vi "Set Control Bounds.vi"(0 "Display State In":T2 {"Time_data" format="%<%.3X>T"}, 6 "Container Dimension":T1, 8 "Relative Size":dbl, 9 "Container State":T3, 11 "error in (no error)":errorcluster) -> (4 "Display State Out":T2 {"Time_data" format="%<%.3X>T"}, 15 "error out":errorcluster)   [LabVIEW 2015, in "2D Buffer Display.xctl"]
uses:
  2D Buffer Display.xctl
  <vilib>/_xctls/Container State.ctl
  Graph_State.ctl
  <vilib>/Utility/miscctls.llb/LVBoundsTypeDef.ctl
  <vilib>/_xctls/XControlSupport.lvlib
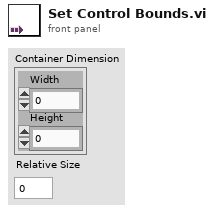
[diagram p1: front panel]
types:
  T1 = typedef "LVBoundsTypeDef.ctl" = cluster{"Width":u32, "Height":u32}
  T2 = typedef "2D Buffer Display.xctl/Graph_State.ctl" = cluster{"History":u16, "Time_data":timestamp[], "Data_Out":sgl[][][], "Channels":bool[], "Variable":bool[], "Variable Tags":string[], "Channel Tags":string[], "Plot Details":cluster{"Name":string, "Line Width":u8, "Line Style":u8, "Color":u32}[], "Y-Axis Labels":string[], "Avg Data":cluster{"mean":dbl, "standard deviation":dbl}[][]}
  T3 = typedef "XControlSupport.lvlib/Container State.ctl" = cluster{"Indicator?":bool, "Run Mode?":bool, " Refnum":refnum<vi>}
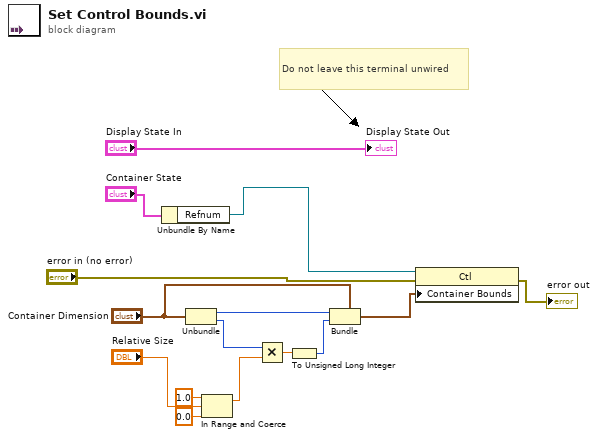
[diagram p0: block diagram]
diagram:
  # "Do not leave this terminal unwired"
  n1 = Unbundle By Name("Container State") -> ("Refnum"=w1:refnum<vi>)
  n2 = Unbundle("Container Dimension") -> ("Width"=w12:u32, "Height"=w11:u32)
  n3 = In Range and Coerce(upper limit=1.0, x="Relative Size", lower limit=0.0) -> (coerced(x)=w2:dbl)  [unwired: 1 out]
  n4 = Multiply(x=w11, y=w2) -> (x*y=w10:dbl)
  n5 = To Unsigned Long Integer(number=w10) -> (unsigned 32bit integer=w9:u32)
  n6 = Bundle(cluster="Container Dimension", "Width"=w12, "Height"=w9) -> (w8:T1)
  n7 = property class="Ctl"(reference=w1, error in="error in (no error)", "Container Bounds"=w8) -> (error out=→"error out":errorcluster)  [unwired: 1 out]
  "Display State Out" <- "Display State In"
